vi "Custom Device CORE.vi"(8 "error in (no error)":errorcluster, 11 "CDW_MetaDataObj":refnum<class "NIVS_Consolidated_CDW_MetaDataObj.lvclass">) -> (0 "error out":errorcluster)   [LabVIEW 2015, in "NIVS_Consolidated_CDW_MetaDataObj.lvclass"]
doc: "This VI is the Core VI for the Custom Device Wizard.\n\nWritten by:\nStephan Daunke\n\nDate:\n2014/01/27\n\nCompany:\nNational Instruments Germany GmbH"
uses:
  NIVS_Consolidated_CDW_MetaDataObj.lvclass
  Action.ctl
  Internal data.ctl
  <resource>/dialog/NewProjectWizard/MetaDataObj/MetaDataObj.lvclass/MetaDataObj.ctl
  NIVS_Consolidated_CDW_MetaDataObj.lvclass/NIVS_Consolidated_CDW_MetaDataObj.ctl
  Template Classes/NIVS_CD Template/NIVS_CD Template.lvclass/NIVS_CD Template.ctl
  Utility folder.ctl
  CD Shared lvlib.ctl
  Common.ctl
  Add Item - Type.ctl
  CD System Explorer lvlib.ctl
  <vilib>/Utility/traverseref.llb/TRef TravTarget.ctl
  CD Engine lvlib.ctl
  Build Spec System Explorer.ctl
  Build Spec Engine.ctl
  <resource>/dialog/NewProjectWizard/MetaDataObj/Accessors/Read Project Root.vi
  Read CD Template.vi
  Template Classes/NIVS_CD Template/Read Extra Page Names.vi
  <resource>/dialog/NewProjectWizard/MetaDataObj/Accessors/Read Project Name.vi
  Utility folder.vi
  CD Shared lvlib.vi
  Common.vi
  CD System Explorer lvlib.vi
  CD Engine lvlib.vi
  <vilib>/Utility/config.llb/Write Key (String).vi
  <vilib>/Utility/config.llb/Write Key (Path).vi
  Build Spec System Explorer.vi
  Build Spec Engine.vi
  Template Classes/NIVS_CD Template/NIVS_CD Template.lvclass
  <vilib>/Utility/config.llb/NI_LVConfig.lvlib
  <vilib>/Utility/Data Type/NI_Data Type.lvlib
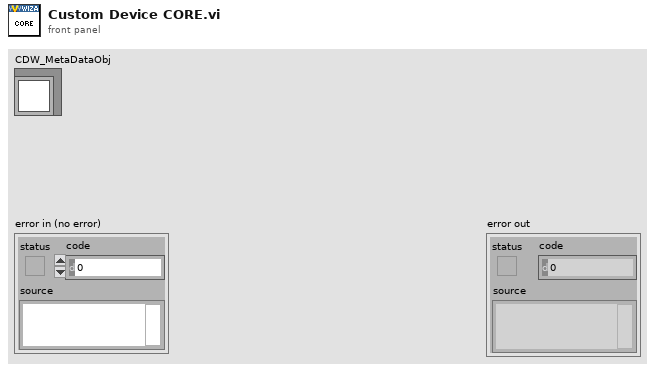
[diagram p1: front panel]
types:
  T1 = typedef "NIVS_Consolidated_CDW_MetaDataObj.lvclass/Internal data.ctl" = cluster{"CD GUID":string, "Extra Page GUIDs":string[], "System Explorer Library":refnum<vi>, "Shared Library":refnum<vi>, "Engine Library":refnum<vi>}
  T2 = typedef "NIVS_Consolidated_CDW_MetaDataObj.lvclass/Action.ctl" = enum16{"Project - Create Custom Device folder", "PC - Create GUID for each extra page", "PC-Utility - Create folder and copy -Copy .LLB to NI VeriStand dir-", "PC-Utility - Change -Copy .LLB to NI VeriStand dir-", "PC-Shared - Create folder and copy Constants.vi", "PC-Shared - Change Constants.vi content", "PC-Shared - Create library", "PC-Shared - Add folders and VIs to library", "PC-System Explorer - Create folder and copy templates", "PC-System Explorer - Create extra pages", "PC-System Explorer - Create library", "PC-System Explorer - Add folders and VIs to library", "PC-Engine - Create folder and copy the RT Template", "PC-Engine - Create library", "PC-Engine - Add virtual folders and VIs to library", "PC-XML - Create and change file", "PC-Help - Copy HTML Files", "Project - Read project file content", "Project - Edit Utility section", "Project - Edit XML section", "Project - Edit Engine Library section", "Project - Edit Shared Library section", "Project - Edit System Explorer Library section", "Project - Edit Custom Device Name", "Project - Edit System Explorer LLB Name", "Project - Edit Engine LLB OS dependent file name", "Project - Write new project file"}
  T3 = typedef "NIVS_Consolidated_CDW_MetaDataObj.lvclass/Utility folder.ctl" = enum16{"Utility.FolderName", "Utility.Copy .llb to NI VeriStand dir.FileName", "Utility.Copy .llb to NI VeriStand dir.FilePathAndName", "Utility.LLB Pre Build.FilePathAndName"}
  T4 = typedef "NIVS_Consolidated_CDW_MetaDataObj.lvclass/CD Shared lvlib.ctl" = enum16{"LibraryFileName", "LibraryFolderName", "ConstantsVI.VIPathAndName", "Shared.FolderName", "Shared.Types.FolderName", "Shared.Constants.VIName", "Shared.Constants.VITemplateName", "Shared.Constants.VITemplatePathAndName", "Shared.CompiledSettings.RelativePath", "Shared.Constants.RelativePath", "Shared.CompiledSettings.Name", "Shared.CompiledSettings.Name.NoExtension", "Shared.CompiledSettings.ClusterName"}
  T5 = typedef "NIVS_Consolidated_CDW_MetaDataObj.lvclass/Common.ctl" = enum16{"ProjectName", "TemplatesFolderName", "ProjectTemplatePathAndName", "TimingAndSyncFolderName", "CustomDeviceFolderName", "PathToTemplates"}
  T6 = typedef "NIVS_Consolidated_CDW_MetaDataObj.lvclass/Add Item - Type.ctl" = string
  T7 = typedef "NIVS_Consolidated_CDW_MetaDataObj.lvclass/CD System Explorer lvlib.ctl" = enum16{"LibraryFileName", "LibraryFolderName", "System Explorer.FolderName", "System Explorer.Dynamically Called.FolderName", "System Explorer.Dynamically Called.Extra Pages.FolderName", "System Explorer.Dynamically Called.Extra Pages.TemplatePathAndName", "System Explorer.Dynamically Called.Main Page.VIName", "System Explorer.Dynamically Called.Main Page.TemplatePathAndName", "System Explorer.Dynamically Called.Initialization VI.VIName", "System Explorer.Dynamically Called.Initialization VI.TemplatePathAndName", "System Explorer.SubVI.FolderName", "System Explorer.Types.FolderName", "System Explorer.ActionVIOnCompile.VIName", "System Explorer.ExportConfigRTM.VIName", "System Explorer.LoadHelpFile.VIName"}
  T8 = typedef "TRef TravTarget.ctl" = enum16{"FP", "BD", "Other"}
  T9 = typedef "NIVS_Consolidated_CDW_MetaDataObj.lvclass/CD Engine lvlib.ctl" = enum16{"LibraryFileName", "LibraryFolderName", "Engine.FolderName", "Engine.Init.FolderName", "Engine.Run.FolderName", "Engine.Shutdown.FolderName", "Types.FolderName", "Engine.RT Driver VI.TemplatePath", "Engine.RT Driver VI.FileName", "Engine.RTStateVariables.Name", "Engine.RTStateVariables.Name.NoExtension", "Engine.Async.NameExtension", "Engine.Async.TemplateName"}
  T10 = typedef "NIVS_Consolidated_CDW_MetaDataObj.lvclass/Build Spec System Explorer.ctl" = enum16{"Destinations.LLBFileName"}
  T11 = typedef "NIVS_Consolidated_CDW_MetaDataObj.lvclass/Build Spec Engine.ctl" = enum16{"Destinations.LLBWindowsFileName", "Destinations.LLBVxWorksFileName", "Destinations.LLBPharlapFileName", "Destinations.LLBLinuxARMFileName", "Destinations.LLBLinux64FileName"}
  T12 = enum16{"open", "replace", "create", "open or create", "replace or create", "replace or create with confirmation"}
  T13 = typedef "NI_LVConfig.lvlib/Config Data RefNum.ctl" = refnum<k1>
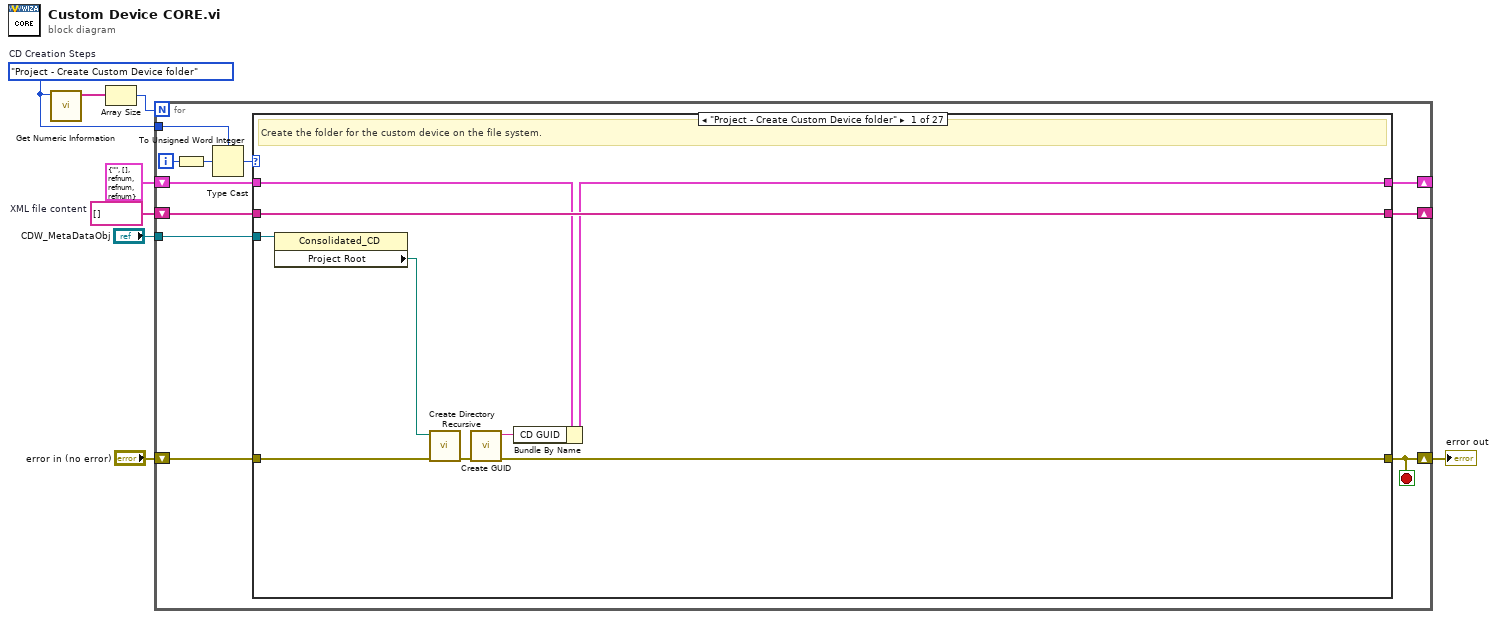
[diagram p0: block diagram]
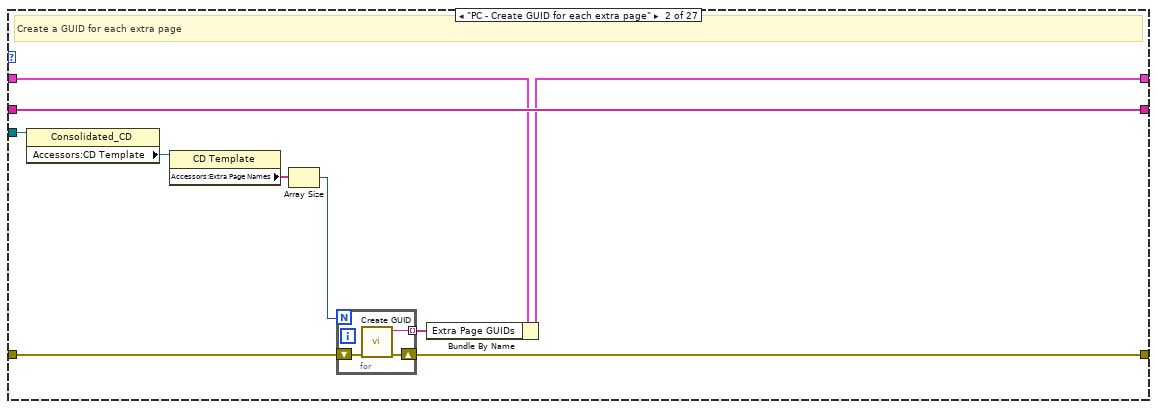
[diagram p2: hidden frame]
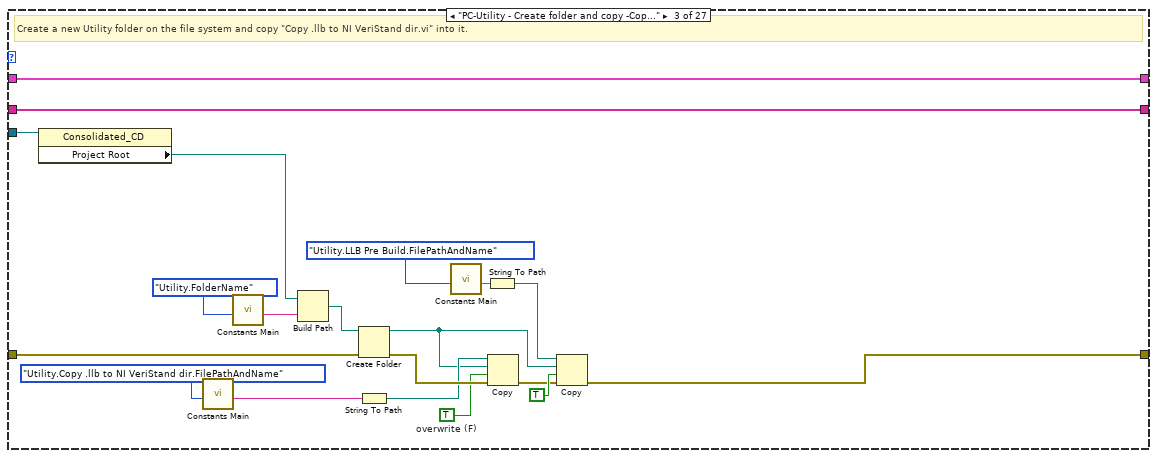
[diagram p3: hidden frame]
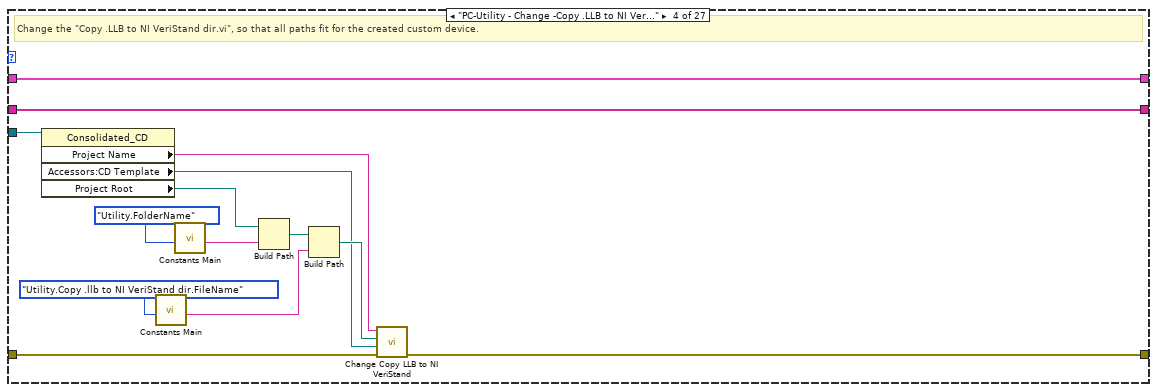
[diagram p4: hidden frame]
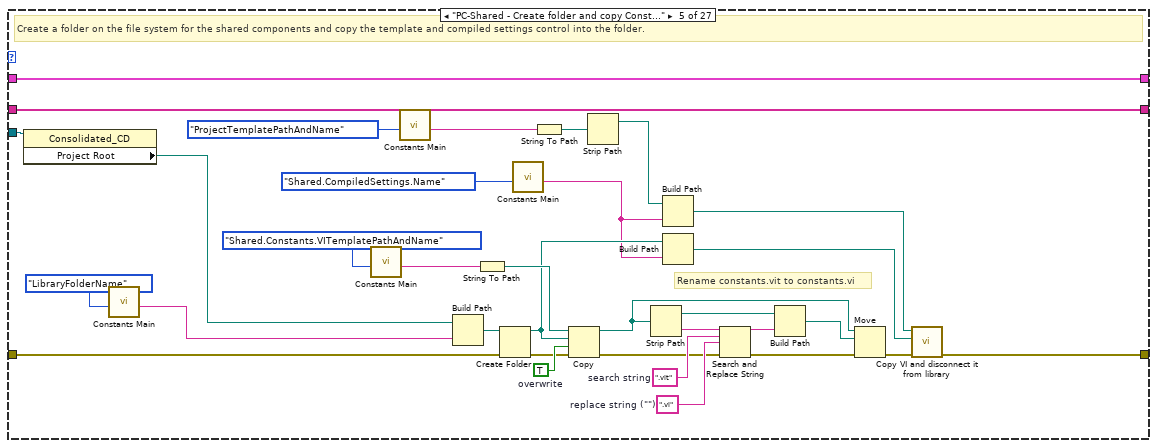
[diagram p5: hidden frame]
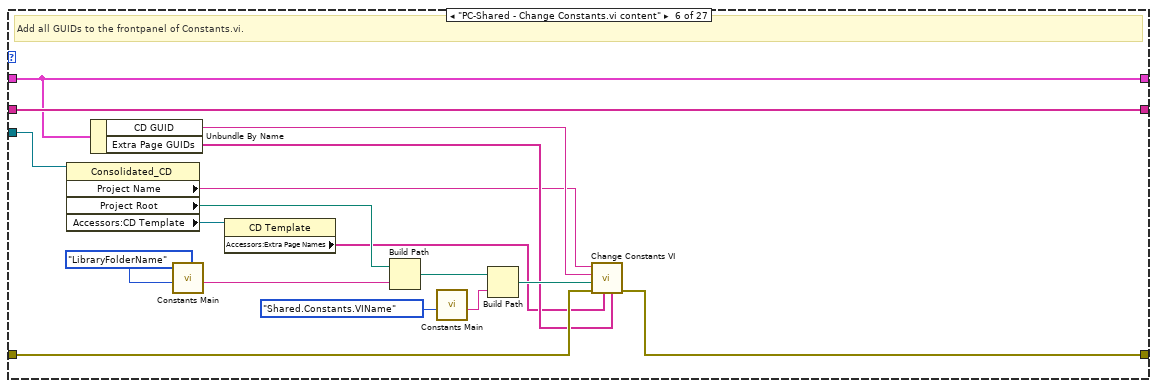
[diagram p6: hidden frame]
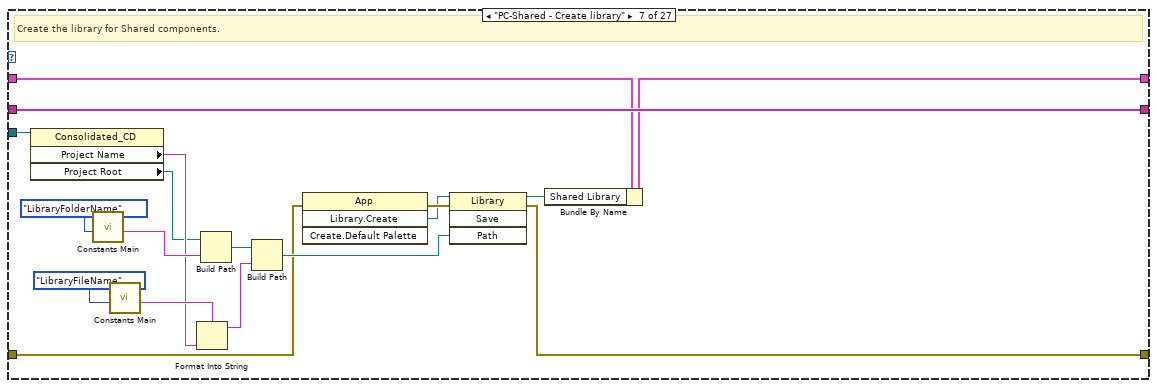
[diagram p7: hidden frame]
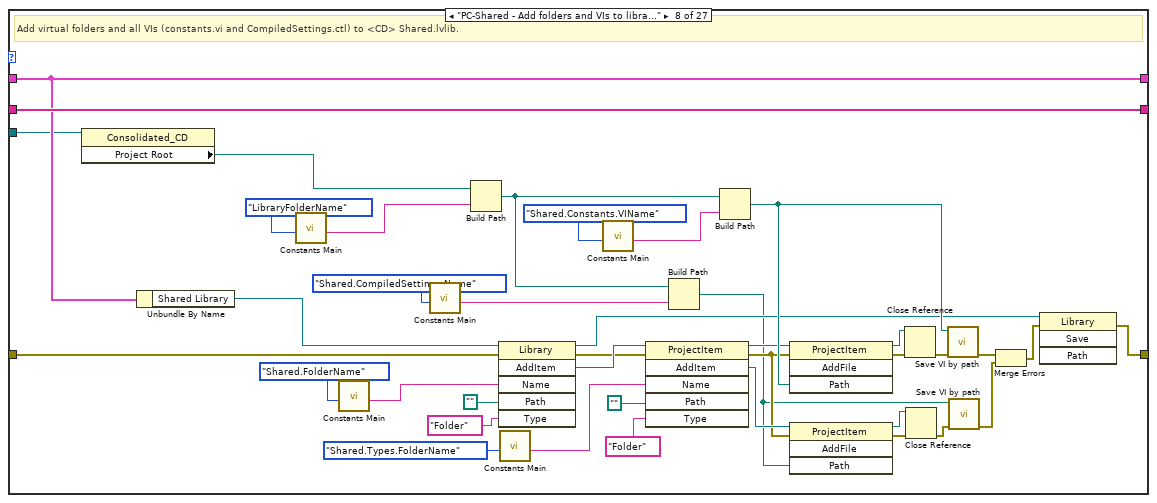
[diagram p8: hidden frame]
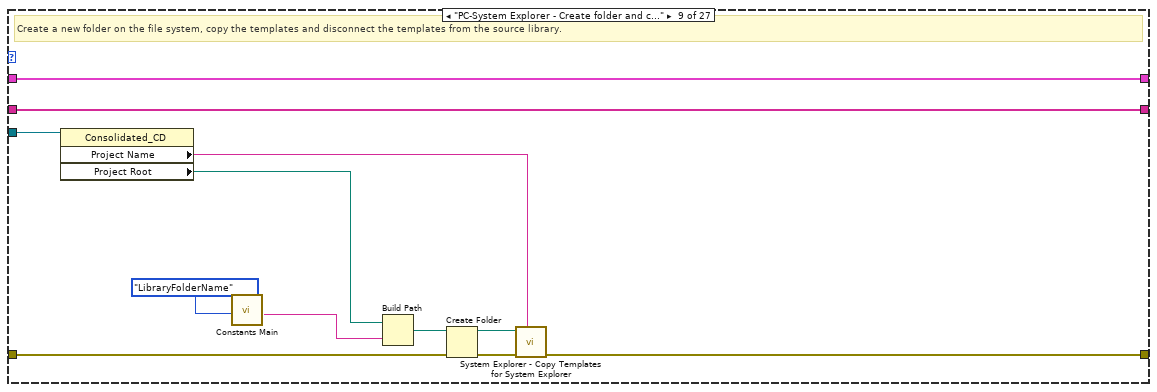
[diagram p9: hidden frame]
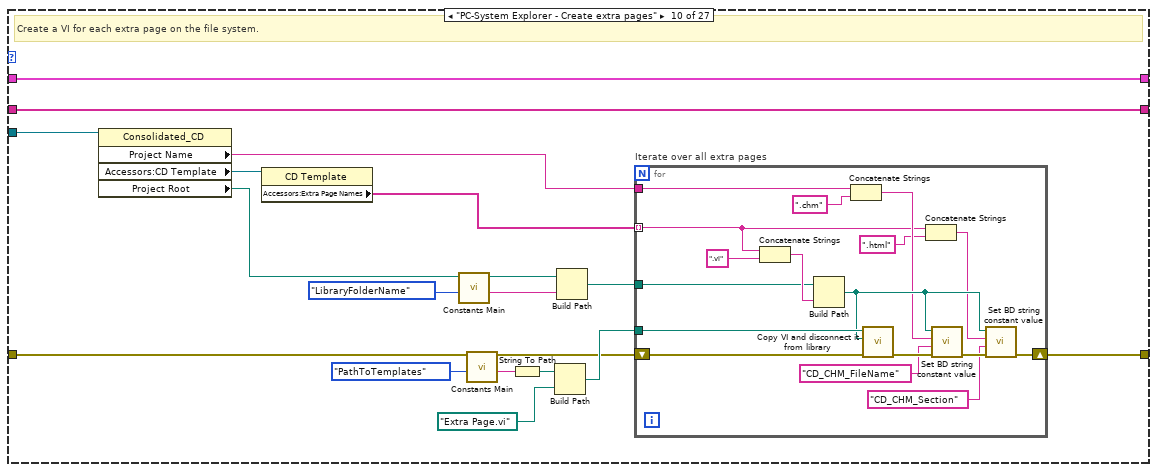
[diagram p10: hidden frame]
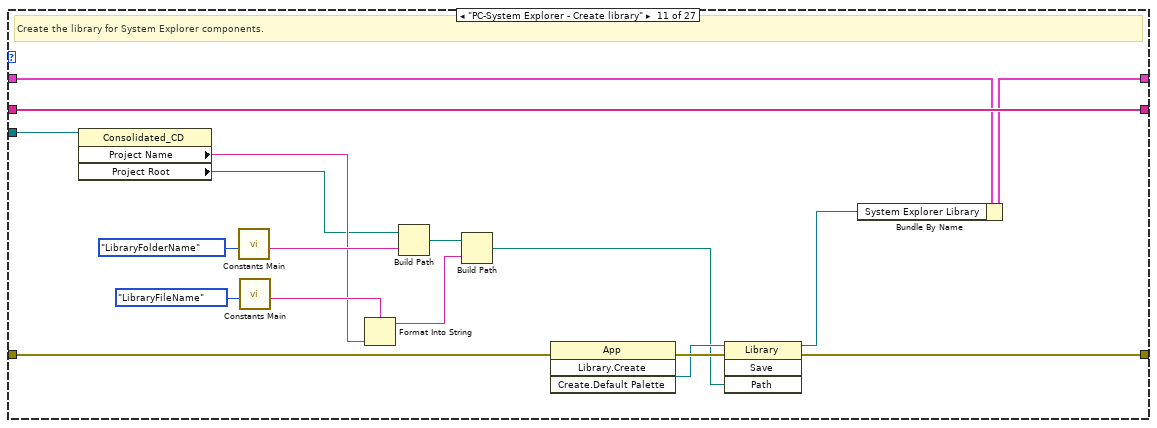
[diagram p11: hidden frame]
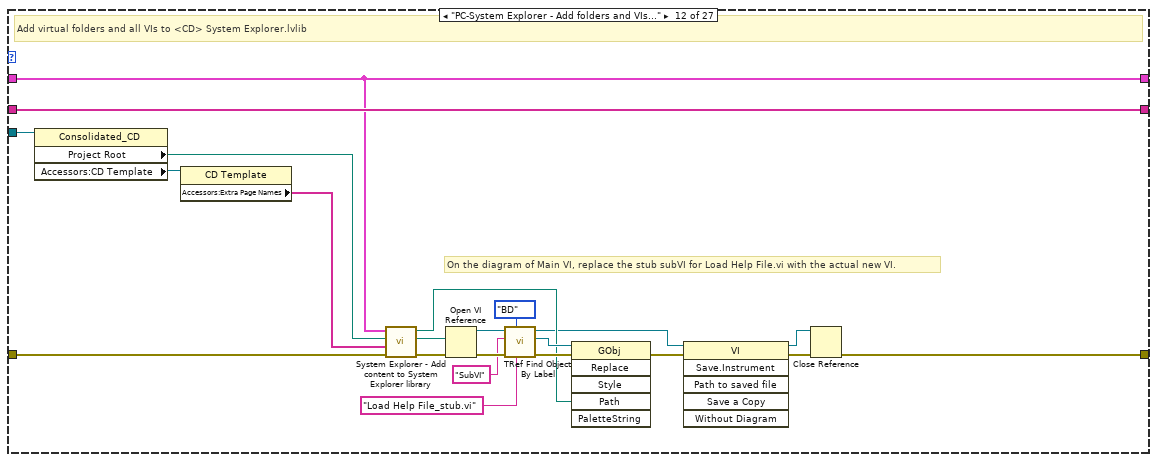
[diagram p12: hidden frame]
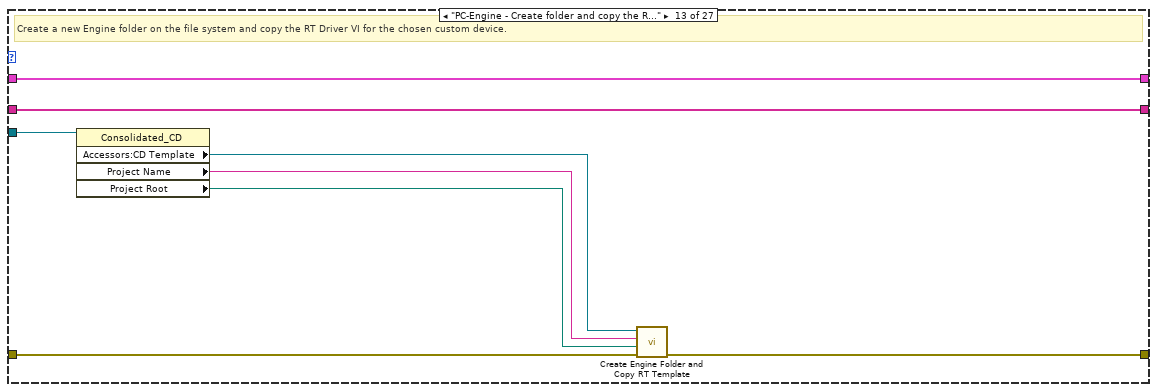
[diagram p13: hidden frame]
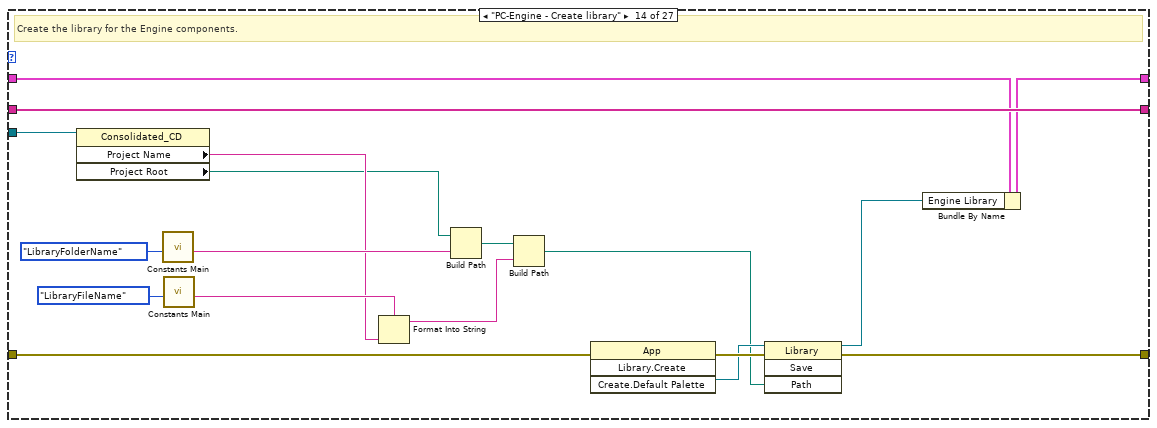
[diagram p14: hidden frame]
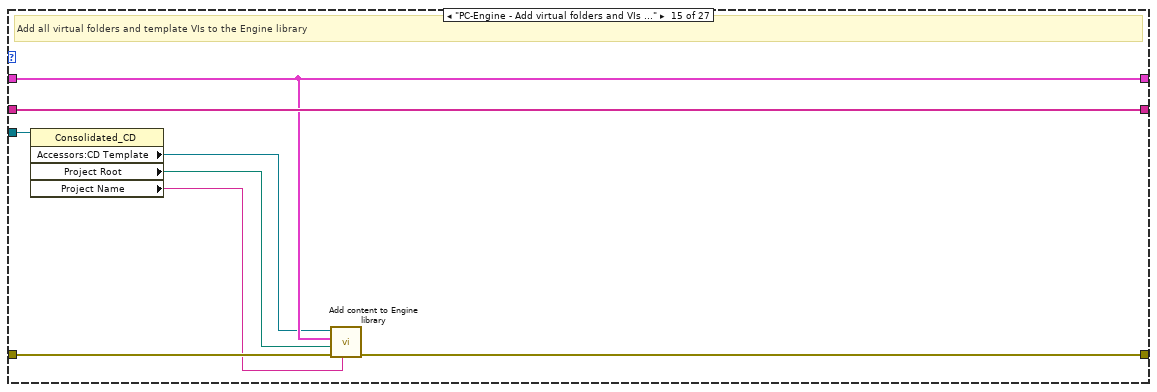
[diagram p15: hidden frame]
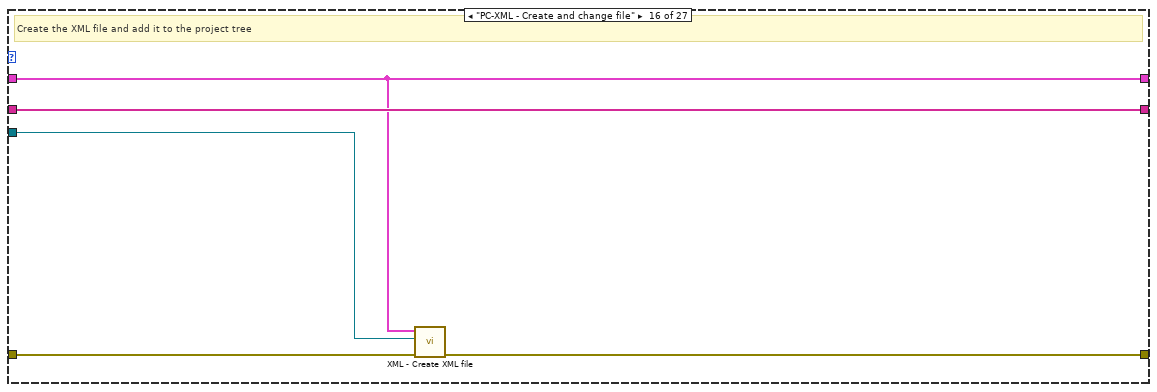
[diagram p16: hidden frame]
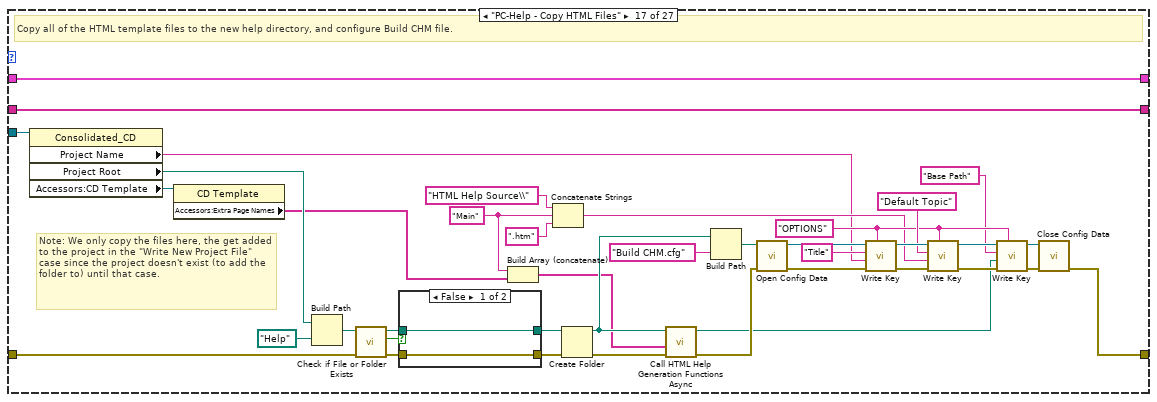
[diagram p17: hidden frame]
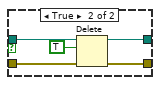
[diagram p18: hidden frame]
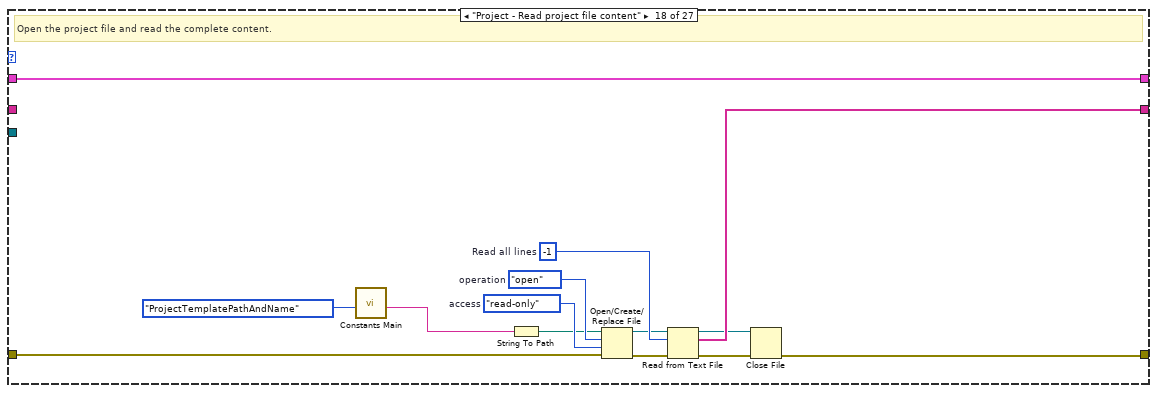
[diagram p19: hidden frame]
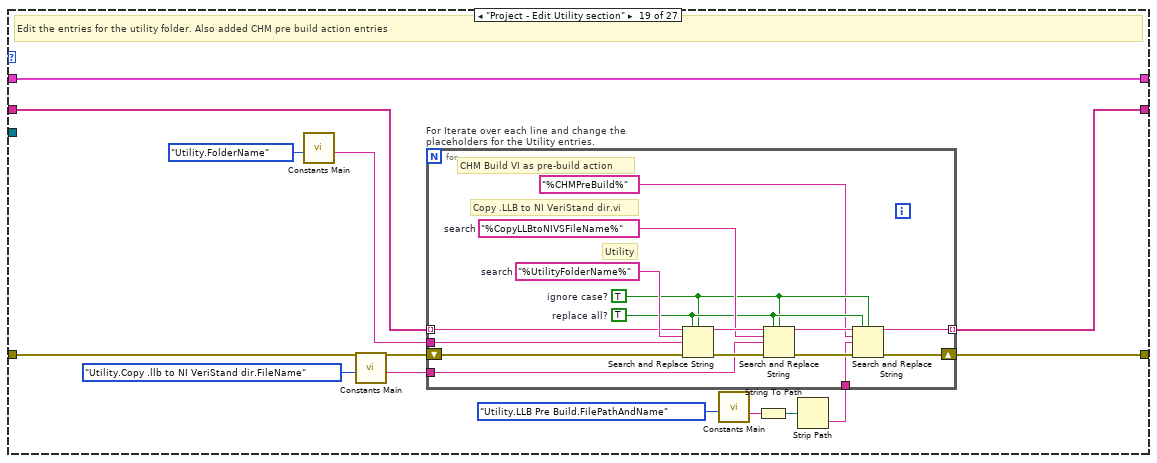
[diagram p20: hidden frame]
diagram:
  w4 = Action."Project - Create Custom Device folder"  # CD Creation Steps
  w5 = string[] []  # XML file content
  n1 = call <vilib>:"Get Numeric Information.vi"("Variant"=w4) -> ("Enum Names"=w3:string[])  [unwired: 7 in, 3 out]
  n2 = Array Size(array=w3) -> (size(s)=w2:i32)
  n3 = for {
    N: w2 -> [_]
    shift-right: [w16] -> _
    shift-left: T1 {"CD GUID"="", "Extra Page GUIDs"=[], "System Explorer Library"=refnum, "Shared Library"=refnum, "Engine Library"=refnum} ("CD Wizard - Internal Data") -> [w18]
    shift-right: [w15] -> _
    shift-left: w5 -> [w17]
    shift-right: [w14] -> w6
    shift-left: "error in (no error)" -> [w19]
    tunnel: w4 -> [w12]
    tunnel: "CDW_MetaDataObj" -> [w11]
    i -> [w13]
    stop <- w14 stop-if-true
    n4 = To Unsigned Word Integer(number=w13) -> (unsigned 16bit integer=w9:u16)
    n5 = Type Cast(type=w12, x=w9) -> (*(type *) &x=w10:T2)
    n6 = case shown="\"Project - Create Custom Device folder\"" w10 {
      tunnel: w19 -> [w24 w37 w43 w63 w78 w118 w129 w145 w183 w200 w232 w267 w275 w280 w301 w306 w324 w354 w367 w399 w418 w422 w452 w486 w497 w515 w553]
      tunnel: [w25 w36 w47 w69 w80 w124 w130 w163 w188 w210 w233 w252 w274 w283 w300 w305 w323 w360 w376 w404 w417 w432 w456 w485 w504 w527 w560] -> w14
      tunnel: w18 -> [w22 w34 w46 w67 w79 w115 w133 w164 w187 w209 w238 w265 w273 w287 w298 w304 w319 w366 w379 w401 w416 w423 w453 w482 w501 w533 w585]
      tunnel: w17 -> [w28 w38 w61 w75 w108 w125 w143 w182 w194 w211 w246 w268 w276 w294 w302 w307 w346 _ w378 w403 w415 w427 w454 w483 w499 w528 w579]
      tunnel: [w27 w33 w46 w67 w79 w115 w132 w164 w187 w209 w239 w265 w273 w286 w298 w304 w319 w366 w379 w401 w416 w423 w453 w482 w501 w533 w585] -> w16
      tunnel: [w28 w38 w61 w75 w108 w125 w143 w182 w194 w211 w246 w268 w276 w294 w302 w307 w346 w359 w377 w402 w419 w433 w455 w484 w498 w516 w579] -> w15
      tunnel: w11 -> [w21 w32 w45 w66 w77 w117 w128 w147 w186 w199 w231 w250 w272 w279 w299 w303 w312 _ _ w398 w414 w421 w451 w481 w496 w514 w552]
      frame "Project - Create Custom Device folder" {
        # "Create the folder for the custom device on the file system."
        n7 = property class="Consolidated_CD"(reference=w21) -> ("Project Root"=w20:path)  [unwired: 1 in, 2 out]
        n8 = call <vilib>:"Create Directory Recursive.vi"("error in (no error)"=w24, "directory"=w20) -> ("error out"=w23:errorcluster)  [unwired: 3 in, 2 out]
        n9 = call "Create GUID.vi"("error in (no error)"=w23) -> ("error out"=w25:errorcluster, "Generated GUID"=w26:string)  [unwired: 9 in]
        n10 = Bundle By Name(cluster=w22, "CD GUID"=w26) -> (w27:T1)
      }
      frame "PC - Create GUID for each extra page" {
        # "Create a GUID for each extra page"
        n11 = property class="Consolidated_CD"(reference=w32) -> ("Accessors:CD Template"=w31:refnum<class "NIVS_CD Template.lvclass">)  [unwired: 1 in, 2 out]
        n12 = property class="CD Template"(reference=w31) -> ("Accessors:Extra Page Names"=w30:string[])  [unwired: 1 in, 2 out]
        n13 = Array Size(array=w30) -> (size(s)=w29:i32)
        n14 = for {
          N: w29 -> [_]
          shift-right: [w40] -> w36
          shift-left: w37 -> [w41]
          tunnel: [w39] -> w35 mode=indexing
          n15 = call "Create GUID.vi"("error in (no error)"=w41) -> ("error out"=w40:errorcluster, "Generated GUID"=w39:string)  [unwired: 9 in]
        }
        n16 = Bundle By Name(cluster=w34, "Extra Page GUIDs"=w35) -> (w33:T1)
      }
      frame "PC-Utility - Create folder and copy -Copy .LLB to NI VeriStand dir-" {
        w58 = TRUE  # overwrite (F)
        # "Create a new Utility folder on the file system and copy \"Copy .llb to NI VeriStand dir.vi\" into it."
        n17 = property class="Consolidated_CD"(reference=w45) -> ("Project Root"=w44:path)  [unwired: 1 in, 2 out]
        n18 = call-poly "Constants Main.vi"("Action"=Utility_folder."Utility.Copy .llb to NI VeriStand dir.FilePathAndName") -> ("Output"=w56:string)  [unwired: 10 in]
        n19 = call-poly "Constants Main.vi"("Action"=Utility_folder."Utility.FolderName") -> ("Output"=w53:string)  [unwired: 10 in]
        n20 = Build Path(base path=w44, name or relative path=w53) -> (appended path=w60:path)
        n21 = Create Folder(path (use dialog)=w60, error in=w43) -> (created path=w52:path, error out=w59:errorcluster)  [unwired: 1 in, 1 out]
        n22 = String To Path(string=w56) -> (path=w55:path)
        n23 = call-poly "Constants Main.vi"("Action"=Utility_folder."Utility.LLB Pre Build.FilePathAndName") -> ("Output"=w50:string)  [unwired: 10 in]
        n24 = String To Path(string=w50) -> (path=w49:path)
        n25 = Copy(8:w59, 9:w58, 10:w52, 11:w55) -> (0:w42:errorcluster)  [unwired: 3 out]
        n26 = Copy(8:w42, 9:TRUE ("overwrite (F)"), 10:w52, 11:w49) -> (0:w47:errorcluster)  [unwired: 3 out]
      }
      frame "PC-Utility - Change -Copy .LLB to NI VeriStand dir-" {
        # "Change the \"Copy .LLB to NI VeriStand dir.vi\", so that all paths fit for the created custom device."
        n27 = property class="Consolidated_CD"(reference=w66) -> ("Project Name"=w65:string, "Accessors:CD Template"=w64:refnum<class "NIVS_CD Template.lvclass">, "Project Root"=w62:path)  [unwired: 1 in, 2 out]
        n28 = call-poly "Constants Main.vi"("Action"=Utility_folder."Utility.Copy .llb to NI VeriStand dir.FileName") -> ("Output"=w70:string)  [unwired: 10 in]
        n29 = call-poly "Constants Main.vi"("Action"=Utility_folder."Utility.FolderName") -> ("Output"=w72:string)  [unwired: 10 in]
        n30 = Build Path(base path=w62, name or relative path=w72) -> (appended path=w71:path)
        n31 = Build Path(base path=w71, name or relative path=w70) -> (appended path=w68:path)
        n32 = call "Change Copy LLB to NI VeriStand.vi"("error in (no error)"=w63, "CD Template"=w64, "Copy .LLB to ... path"=w68, "CD Name"=w65) -> ("error out"=w69:errorcluster)  [unwired: 7 in]
      }
      frame "PC-Shared - Create folder and copy Constants.vi" {
        w97 = ".vi"  # replace string ("")
        w98 = ".vit"  # search string
        w102 = TRUE  # overwrite
        # "Rename constants.vit to constants.vi"
        # "Create a folder on the file system for the shared components and copy the template and compiled settings control into the folder."
        n33 = property class="Consolidated_CD"(reference=w77) -> ("Project Root"=w76:path)  [unwired: 1 in, 2 out]
        n34 = call-poly "Constants Main.vi"("Action"=CD_Shared_lvlib."LibraryFolderName") -> ("Output"=w105:string)  [unwired: 10 in]
        n35 = call-poly "Constants Main.vi"("Action"=CD_Shared_lvlib."Shared.Constants.VITemplatePathAndName") -> ("Output"=w103:string)  [unwired: 10 in]
        n36 = call-poly "Constants Main.vi"("Action"=Common."ProjectTemplatePathAndName") -> ("Output"=w89:string)  [unwired: 10 in]
        n37 = Build Path(base path=w76, name or relative path=w105) -> (appended path=w107:path)
        n38 = String To Path(string=w103) -> (path=w95:path)
        n39 = Create Folder(path (use dialog)=w107, error in=w78) -> (created path=w86:path, error out=w96:errorcluster)  [unwired: 1 in, 1 out]
        n40 = call-poly "Constants Main.vi"("Action"=CD_Shared_lvlib."Shared.CompiledSettings.Name") -> ("Output"=w81:string)  [unwired: 10 in]
        n41 = String To Path(string=w89) -> (path=w88:path)
        n42 = Copy(8:w96, 9:w102, 10:w86, 11:w95) -> (0:w94:errorcluster, 3:w91:path)  [unwired: 2 out]
        n43 = Strip Path(path=w88) -> (stripped path=w87:path)  [unwired: 1 out]
        n44 = Strip Path(path=w91) -> (stripped path=w101:path, name=w100:string)
        n45 = Build Path(base path=w87, name or relative path=w81) -> (appended path=w85:path)
        n46 = Build Path(base path=w86, name or relative path=w81) -> (appended path=w84:path)
        n47 = Search and Replace String(input string=w100, search string=w98, replace string=w97, error in=w94) -> (result string=w99:string, error out=w93:errorcluster)  [unwired: 4 in, 2 out]
        n48 = Build Path(base path=w101, name or relative path=w99) -> (appended path=w92:path)
        n49 = Move(source path=w91, error in=w93, 10:w92) -> (error out=w83:errorcluster)  [unwired: 2 in, 2 out]
        n50 = call "Copy VI and disconnect it from library.vi"("error in (no error)"=w83, "VI Target Path"=w84, "VI Source Path"=w85) -> ("error out"=w80:errorcluster)  [unwired: 8 in]
      }
      frame "PC-Shared - Change Constants.vi content" {
        # "Add all GUIDs to the frontpanel of Constants.vi."
        n51 = property class="Consolidated_CD"(reference=w117) -> ("Project Name"=w111:string, "Project Root"=w116:path, "Accessors:CD Template"=w110:refnum<class "NIVS_CD Template.lvclass">)  [unwired: 1 in, 2 out]
        n52 = Unbundle By Name(w115) -> ("CD GUID"=w113:string, "Extra Page GUIDs"=w112:string[])
        n53 = call-poly "Constants Main.vi"("Action"=CD_Shared_lvlib."LibraryFolderName") -> ("Output"=w119:string)  [unwired: 10 in]
        n54 = property class="CD Template"(reference=w110) -> ("Accessors:Extra Page Names"=w109:string[])  [unwired: 1 in, 2 out]
        n55 = Build Path(base path=w116, name or relative path=w119) -> (appended path=w123:path)
        n56 = call-poly "Constants Main.vi"("Action"=CD_Shared_lvlib."Shared.Constants.VIName") -> ("Output"=w121:string)  [unwired: 10 in]
        n57 = Build Path(base path=w123, name or relative path=w121) -> (appended path=w114:path)
        n58 = call "Change Constants VI.vi"("Extra Page GUIDs"=w112, "Extra Page Names"=w109, "error in (no error)"=w118, "Constants.vi path"=w114, "CD GUID"=w113, "CD Name"=w111) -> ("error out"=w124:errorcluster)  [unwired: 5 in]
      }
      frame "PC-Shared - Create library" {
        # "Create the library for Shared components."
        n59 = property class="Consolidated_CD"(reference=w128) -> ("Project Name"=w127:string, "Project Root"=w126:path)  [unwired: 1 in, 2 out]
        n60 = call-poly "Constants Main.vi"("Action"=CD_Shared_lvlib."LibraryFolderName") -> ("Output"=w137:string)  [unwired: 10 in]
        n61 = call-poly "Constants Main.vi"("Action"=CD_Shared_lvlib."LibraryFileName") -> ("Output"=w138:string)  [unwired: 10 in]
        n62 = Format Into String(format string=w138, w127) -> (resulting string=w141:string)  [unwired: 2 in, 1 out]
        n63 = Build Path(base path=w126, name or relative path=w137) -> (appended path=w142:path)
        n64 = Build Path(base path=w142, name or relative path=w141) -> (appended path=w134:path)
        n65 = invoke class="App" method="Library.Create"(error in=w129) -> (error out=w136:errorcluster, "Create Library"=w135:refnum<vi>)  [unwired: 3 in, 2 out]
        n66 = invoke class="Library" method="Save"(reference=w135, error in=w136, "Path"=w134) -> (reference out=w131:refnum<vi>, error out=w130:errorcluster)  [unwired: 1 in, 2 out]
        n67 = Bundle By Name(cluster=w133, "Shared Library"=w131) -> (w132:T1)
      }
      frame "PC-Shared - Add folders and VIs to library" {
        # "Add virtual folders and all VIs (constants.vi and CompiledSettings.ctl) to <CD> Shared.lvlib."
        n68 = property class="Consolidated_CD"(reference=w147) -> ("Project Root"=w146:path)  [unwired: 1 in, 2 out]
        n69 = Unbundle By Name(w164) -> ("Shared Library"=w166:refnum<vi>)
        n70 = call-poly "Constants Main.vi"("Action"=CD_Shared_lvlib."LibraryFolderName") -> ("Output"=w160:string)  [unwired: 10 in]
        n71 = call-poly "Constants Main.vi"("Action"=CD_Shared_lvlib."Shared.FolderName") -> ("Output"=w161:string)  [unwired: 10 in]
        n72 = call-poly "Constants Main.vi"("Action"=CD_Shared_lvlib."Shared.CompiledSettings.Name") -> ("Output"=w152:string)  [unwired: 10 in]
        n73 = Build Path(base path=w146, name or relative path=w160) -> (appended path=w157:path)
        n74 = invoke class="Library" method="AddItem"(reference=w166, error in=w145, "Name"=w161, "Path"=path "", "Type"=T6 "Folder" ("Add Item - Type")) -> (reference out=w172:refnum<vi>, error out=w167:errorcluster, "AddItem"=w169:refnum<vi>)  [unwired: 1 in, 3 out]
        n75 = call-poly "Constants Main.vi"("Action"=CD_Shared_lvlib."Shared.Types.FolderName") -> ("Output"=w180:string)  [unwired: 10 in]
        n76 = call-poly "Constants Main.vi"("Action"=CD_Shared_lvlib."Shared.Constants.VIName") -> ("Output"=w148:string)  [unwired: 10 in]
        n77 = invoke class="ProjectItem" method="AddItem"(reference=w169, error in=w167, "Name"=w180, "Path"=path "", "Type"=T6 "Folder" ("Add Item - Type")) -> (reference out=w171:refnum<vi>, error out=w158:errorcluster, "AddItem"=w159:refnum<vi>)  [unwired: 1 in, 3 out]
        n78 = Build Path(base path=w157, name or relative path=w152) -> (appended path=w156:path)
        n79 = Build Path(base path=w157, name or relative path=w148) -> (appended path=w173:path)
        n80 = invoke class="ProjectItem" method="AddFile"(reference=w171, error in=w158, "Path"=w173) -> (reference out=w176:refnum<vi>, error out=w175:errorcluster)  [unwired: 1 in, 2 out]
        n81 = invoke class="ProjectItem" method="AddFile"(reference=w159, error in=w158, "Path"=w156) -> (reference out=w150:refnum<vi>, error out=w149:errorcluster)  [unwired: 1 in, 2 out]
        n82 = Close Reference(reference=w176, error in (no error)=w175) -> (error out=w177:errorcluster)
        n83 = Close Reference(reference=w150, error in (no error)=w149) -> (error out=w151:errorcluster)
        n84 = call "Save VI by path.vi"("error in (no error)"=w177, "VI path"=w173) -> ("error out"=w174:errorcluster)  [unwired: 9 in]
        n85 = call "Save VI by path.vi"("error in (no error)"=w151, "VI path"=w156) -> ("error out"=w154:errorcluster)  [unwired: 9 in]
        n86 = Merge Errors(w174, w154) -> (w155:errorcluster)
        n87 = invoke class="Library" method="Save"(reference=w172, error in=w155) -> (error out=w163:errorcluster)  [unwired: 2 in, 3 out]
      }
      frame "PC-System Explorer - Create folder and copy templates" {
        # "Create a new folder on the file system, copy the templates and disconnect the templates from the source library."
        n88 = property class="Consolidated_CD"(reference=w186) -> ("Project Name"=w185:string, "Project Root"=w184:path)  [unwired: 1 in, 2 out]
        n89 = call-poly "Constants Main.vi"("Action"=CD_System_Explorer_lvlib."LibraryFolderName") -> ("Output"=w191:string)  [unwired: 10 in]
        n90 = Build Path(base path=w184, name or relative path=w191) -> (appended path=w193:path)
        n91 = Create Folder(path (use dialog)=w193, error in=w183) -> (created path=w189:path, error out=w190:errorcluster)  [unwired: 1 in, 1 out]
        n92 = call "System Explorer - Copy Templates for System Explorer.vi"("CD Name"=w185, "error in (no error)"=w190, "System Explorer folder"=w189) -> ("error out"=w188:errorcluster)  [unwired: 8 in]
      }
      frame "PC-System Explorer - Create extra pages" {
        # "Create a VI for each extra page on the file system."
        n93 = property class="Consolidated_CD"(reference=w199) -> ("Project Name"=w198:string, "Accessors:CD Template"=w197:refnum<class "NIVS_CD Template.lvclass">, "Project Root"=w195:path)  [unwired: 1 in, 2 out]
        n94 = property class="CD Template"(reference=w197) -> ("Accessors:Extra Page Names"=w196:string[])  [unwired: 1 in, 2 out]
        n95 = call-poly "Constants Main.vi"("Action"=CD_System_Explorer_lvlib."LibraryFolderName") -> ("Output"=w207:string)  [unwired: 10 in]
        n96 = call-poly "Constants Main.vi"("Action"=Common."PathToTemplates") -> ("Output"=w203:string)  [unwired: 10 in]
        n97 = String To Path(string=w203) -> (path=w202:path)
        n98 = Build Path(base path=w202, name or relative path=path "Extra Page.vi") -> (appended path=w208:path)
        n99 = Build Path(base path=w195, name or relative path=w207) -> (appended path=w205:path)
        n100 = for "Iterate over all extra pages" {
          tunnel: w196 -> [w212] mode=indexing
          shift-right: [w217] -> w210
          shift-left: w200 -> [w226]
          tunnel: w205 -> [w224]
          tunnel: w208 -> [w225]
          tunnel: w198 -> [w221]
          n101 = Concatenate Strings(w212, ".vi") -> (w227:string)
          n102 = Build Path(base path=w224, name or relative path=w227) -> (appended path=w219:path)
          n103 = Concatenate Strings(w221, ".chm" ("string")) -> (w216:string)
          n104 = call "Copy VI and disconnect it from library.vi"("error in (no error)"=w226, "VI Target Path"=w219, "VI Source Path"=w225) -> ("error out"=w223:errorcluster)  [unwired: 8 in]
          n105 = Concatenate Strings(w212, ".html" ("string")) -> (w214:string)
          n106 = call "Set BD string constant value.vi"("error in (no error)"=w223, "Name of string constant"="CD_CHM_FileName", "New String Value"=w216, "Path to VI"=w219) -> ("error out"=w220:errorcluster)  [unwired: 7 in]
          n107 = call "Set BD string constant value.vi"("error in (no error)"=w220, "Name of string constant"="CD_CHM_Section", "New String Value"=w214, "Path to VI"=w219) -> ("error out"=w217:errorcluster)  [unwired: 7 in]
        }
      }
      frame "PC-System Explorer - Create library" {
        # "Create the library for System Explorer components."
        n108 = property class="Consolidated_CD"(reference=w231) -> ("Project Name"=w230:string, "Project Root"=w229:path)  [unwired: 1 in, 2 out]
        n109 = call-poly "Constants Main.vi"("Action"=CD_System_Explorer_lvlib."LibraryFolderName") -> ("Output"=w242:string)  [unwired: 10 in]
        n110 = call-poly "Constants Main.vi"("Action"=CD_System_Explorer_lvlib."LibraryFileName") -> ("Output"=w243:string)  [unwired: 10 in]
        n111 = Format Into String(format string=w243, w230) -> (resulting string=w244:string)  [unwired: 2 in, 1 out]
        n112 = Build Path(base path=w229, name or relative path=w242) -> (appended path=w245:path)
        n113 = Build Path(base path=w245, name or relative path=w244) -> (appended path=w234:path)
        n114 = invoke class="App" method="Library.Create"(error in=w232) -> (error out=w237:errorcluster, "Create Library"=w236:refnum<vi>)  [unwired: 3 in, 2 out]
        n115 = invoke class="Library" method="Save"(reference=w236, error in=w237, "Path"=w234) -> (reference out=w235:refnum<vi>, error out=w233:errorcluster)  [unwired: 1 in, 2 out]
        n116 = Bundle By Name(cluster=w238, "System Explorer Library"=w235) -> (w239:T1)
      }
      frame "PC-System Explorer - Add folders and VIs to library" {
        # "On the diagram of Main VI, replace the stub subVI for Load Help File.vi with the actual new VI."
        # "Add virtual folders and all VIs to <CD> System Explorer.lvlib"
        n117 = property class="Consolidated_CD"(reference=w250) -> ("Project Root"=w249:path, "Accessors:CD Template"=w248:refnum<class "NIVS_CD Template.lvclass">)  [unwired: 1 in, 2 out]
        n118 = property class="CD Template"(reference=w248) -> ("Accessors:Extra Page Names"=w247:string[])  [unwired: 1 in, 2 out]
        n119 = call "System Explorer - Add content to System Explorer library.vi"("error in (no error)"=w267, "Extra Page Names"=w247, "Project Root"=w249, "CD Wizard - Internal Data"=w265) -> ("error out"=w266:errorcluster, "System Explorer Main VI"=w256:path, "Load Help File VI"=w255:path)  [unwired: 5 in]
        n120 = Open VI Reference(vi path=w256, error in (no error)=w266) -> (vi reference=w262:refnum<vi>, error out=w264:errorcluster)  [unwired: 4 in]
        n121 = call <vilib>:"TRef Find Object By Label.vi"("Label"="Load Help File_stub.vi", "Traverse Target"=TRef_TravTarget."BD", "error in (no error)"=w264, "Class Name"="SubVI", "VI Ref"=w262) -> ("error out"=w263:errorcluster, "Found Obj Ref"=w257:refnum<vi>, "dup VI Ref"=w253:refnum<vi>)  [unwired: 3 in, 1 out]
        n122 = invoke class="GObj" method="Replace"(reference=w257, error in=w263, "Path"=w255) -> (error out=w258:errorcluster)  [unwired: 3 in, 5 out]
        n123 = invoke class="VI" method="Save.Instrument"(reference=w253, error in=w258) -> (reference out=w251:refnum<vi>, error out=w254:errorcluster)  [unwired: 4 in, 4 out]
        n124 = Close Reference(reference=w251, error in (no error)=w254) -> (error out=w252:errorcluster)
      }
      frame "PC-Engine - Create folder and copy the RT Template" {
        # "Create a new Engine folder on the file system and copy the RT Driver VI for the chosen custom device."
        n125 = property class="Consolidated_CD"(reference=w272) -> ("Accessors:CD Template"=w269:refnum<class "NIVS_CD Template.lvclass">, "Project Name"=w271:string, "Project Root"=w270:path)  [unwired: 1 in, 2 out]
        n126 = call-dynamic "Create Engine Folder and Copy RT Template.vi"("error in (no error)"=w275, "Project Root"=w270, "Project Name"=w271, "CD Template"=w269) -> ("error out"=w274:errorcluster)  [unwired: 7 in]
      }
      frame "PC-Engine - Create library" {
        # "Create the library for the Engine components."
        n127 = property class="Consolidated_CD"(reference=w279) -> ("Project Name"=w278:string, "Project Root"=w277:path)  [unwired: 1 in, 2 out]
        n128 = call-poly "Constants Main.vi"("Action"=CD_Engine_lvlib."LibraryFolderName") -> ("Output"=w290:string)  [unwired: 10 in]
        n129 = call-poly "Constants Main.vi"("Action"=CD_Engine_lvlib."LibraryFileName") -> ("Output"=w291:string)  [unwired: 10 in]
        n130 = Format Into String(format string=w291, w278) -> (resulting string=w292:string)  [unwired: 2 in, 1 out]
        n131 = Build Path(base path=w277, name or relative path=w290) -> (appended path=w293:path)
        n132 = Build Path(base path=w293, name or relative path=w292) -> (appended path=w281:path)
        n133 = invoke class="App" method="Library.Create"(error in=w280) -> (error out=w285:errorcluster, "Create Library"=w284:refnum<vi>)  [unwired: 3 in, 2 out]
        n134 = invoke class="Library" method="Save"(reference=w284, error in=w285, "Path"=w281) -> (reference out=w282:refnum<vi>, error out=w283:errorcluster)  [unwired: 1 in, 2 out]
        n135 = Bundle By Name(cluster=w287, "Engine Library"=w282) -> (w286:T1)
      }
      frame "PC-Engine - Add virtual folders and VIs to library" {
        # "Add all virtual folders and template VIs to the Engine library"
        n136 = property class="Consolidated_CD"(reference=w299) -> ("Accessors:CD Template"=w297:refnum<class "NIVS_CD Template.lvclass">, "Project Root"=w296:path, "Project Name"=w295:string)  [unwired: 1 in, 2 out]
        n137 = call-dynamic "Add content to Engine library.vi"("Project Name"=w295, "error in (no error)"=w301, "Project Root"=w296, "CD Wizard - Internal Data"=w298, "CD Template"=w297) -> ("error out"=w300:errorcluster)  [unwired: 6 in]
      }
      frame "PC-XML - Create and change file" {
        # "Create the XML file and add it to the project tree"
        n138 = call "XML - Create XML file.vi"("error in (no error)"=w306, "Consolidated_CD"=w303, "CD Wizard - Internal Data"=w304) -> ("error out"=w305:errorcluster)  [unwired: 7 in, 1 out]
      }
      frame "PC-Help - Copy HTML Files" {
        w322 = "Main"
        w337 = "OPTIONS" ("section")
        # "Note: We only copy the files here, the get added to the project in the \"Write New Project File\" case since the project doesn't exist (to add the folder to) until that case."
        # "Copy all of the HTML template files to the new help directory, and configure Build CHM file."
        n139 = property class="Consolidated_CD"(reference=w312) -> ("Project Name"=w311:string, "Project Root"=w310:path, "Accessors:CD Template"=w309:refnum<class "NIVS_CD Template.lvclass">)  [unwired: 1 in, 2 out]
        n140 = property class="CD Template"(reference=w309) -> ("Accessors:Extra Page Names"=w308:string[])  [unwired: 1 in, 2 out]
        n141 = Build Path(base path=w310, name or relative path=path "Help") -> (appended path=w321:path)
        n142 = call <vilib>:"Check if File or Folder Exists.vi"("error in (no error)"=w324, "path"=w321) -> ("error out"=w330:errorcluster, "file or folder exists?"=w344:bool, "dup path"=w345:path)  [unwired: 7 in]
        n143 = case shown="False" w344 {
          tunnel: w345 -> [w348 w352]
          tunnel: [w348 w351] -> w316
          tunnel: [w347 w350] -> w331
          tunnel: w330 -> [w347 w349]
          frame False {
          }
          frame True {
            n144 = Delete(path (use dialog)=w352, entire hierarchy (F)=TRUE, error in=w349) -> (deleted path=w351:path, error out=w350:errorcluster)  [unwired: 2 in, 1 out]
          }
        }
        n145 = Build Array (concatenate)(w322, w308) -> (w315:string[])
        n146 = Concatenate Strings("HTML Help Source\\" ("string"), w322, ".htm" ("string")) -> (w326:string)
        n147 = Create Folder(path (use dialog)=w316, error in=w331) -> (created path=w318:path, error out=w317:errorcluster)  [unwired: 1 in, 1 out]
        n148 = call "Call HTML Help Generation Functions Async.vi"("error in (no error)"=w317, "Extra Page Names"=w315, "Destination Base Path"=w318) -> ("error out"=w314:errorcluster, "Destination Base Path Out (dup)"=w313:path)  [unwired: 7 in]
        n149 = Build Path(base path=w318, name or relative path="Build CHM.cfg") -> (appended path=w328:path)
        n150 = call <vilib>:"Open Config Data.vi"("error in (no error)"=w314, "configuration file path"=w328) -> ("error out"=w343:errorcluster, "refnum"=w342:T13)  [unwired: 7 in, 1 out]
        n151 = call-poly <vilib>:"Write Key.vi"("section"=w337, "error in (no error)"=w343, "value"=w311, "key"="Title", "refnum"=w342) -> ("error out"=w340:errorcluster, "refnum out"=w339:T13)  [unwired: 4 in, 1 out]
        n152 = call-poly <vilib>:"Write Key.vi"("section"=w337, "error in (no error)"=w340, "value"=w326, "key"="Default Topic", "refnum"=w339) -> ("error out"=w336:errorcluster, "refnum out"=w334:T13)  [unwired: 4 in, 1 out]
        n153 = call-poly <vilib>:"Write Key.vi"("section"=w337, "error in (no error)"=w336, "value"=w313, "key"="Base Path", "refnum"=w334) -> ("error out"=w335:errorcluster, "refnum out"=w333:T13)  [unwired: 4 in, 1 out]
        n154 = call <vilib>:"Close Config Data.vi"("error in (no error)"=w335, "refnum"=w333) -> ("error out"=w323:errorcluster)  [unwired: 8 in, 1 out]
      }
      frame "Project - Read project file content" {
        w365 = -1  # Read all lines
        w364 = T12."open"  # operation
        w363 = enum16{"read/write", "read-only", "write-only"}."read-only"  # access
        # "Open the project file and read the complete content."
        n155 = call-poly "Constants Main.vi"("Action"=Common."ProjectTemplatePathAndName") -> ("Output"=w356:string)  [unwired: 10 in]
        n156 = String To Path(string=w356) -> (path=w357:path)
        n157 = Open/Create/Replace File(file path (use dialog)=w357, error in=w354, operation (0:open)=w364, access (0:read/write)=w363) -> (refnum out=w361:refnum<file>, error out=w362:errorcluster)  [unwired: 3 out]
        n158 = Read from Text File(file (use dialog)=w361, count=w365, error in=w362) -> (refnum out=w355:refnum<file>, text=w359:string[], error out=w360:errorcluster)  [unwired: 2 out]
        n159 = Close File(refnum=w355) -> ()  [unwired: 1 in, 2 out]
      }
      frame "Project - Edit Utility section" {
        # "Edit the entries for the utility folder. Also added CHM pre build action entries"
        n160 = call-poly "Constants Main.vi"("Action"=Utility_folder."Utility.FolderName") -> ("Output"=w372:string)  [unwired: 10 in]
        n161 = call-poly "Constants Main.vi"("Action"=Utility_folder."Utility.Copy .llb to NI VeriStand dir.FileName") -> ("Output"=w373:string)  [unwired: 10 in]
        n162 = call-poly "Constants Main.vi"("Action"=Utility_folder."Utility.LLB Pre Build.FilePathAndName") -> ("Output"=w370:string)  [unwired: 10 in]
        n163 = String To Path(string=w370) -> (path=w369:path)
        n164 = Strip Path(path=w369) -> (name=w368:string)  [unwired: 1 out]
        n165 = for "For Iterate over each line and change the placeholders for the Utility entries." {
          tunnel: w378 -> [w390] mode=indexing
          shift-right: [w386] -> w376
          shift-left: w367 -> [w388]
          tunnel: [w384] -> w377 mode=indexing
          tunnel: w373 -> [w389]
          tunnel: w372 -> [w387]
          tunnel: w368 -> [w380]
          w382 = TRUE  # ignore case?
          w383 = TRUE  # replace all?
          w393 = "%CopyLLBtoNIVSFileName%"  # search
          w395 = "%UtilityFolderName%"  # search
          # "CHM Build VI as pre-build action"
          # "Copy .LLB to NI VeriStand dir.vi"
          # "Utility"
          n166 = Search and Replace String(replace all?=w383, case sensitive?=w382, input string=w390, search string=w395, replace string=w387, error in=w388) -> (result string=w394:string, error out=w392:errorcluster)  [unwired: 2 in, 2 out]
          n167 = Search and Replace String(replace all?=w383, case sensitive?=w382, input string=w394, search string=w393, replace string=w389, error in=w392) -> (result string=w385:string, error out=w391:errorcluster)  [unwired: 2 in, 2 out]
          n168 = Search and Replace String(replace all?=w383, case sensitive?=w382, input string=w385, search string="%CHMPreBuild%" ("result string"), replace string=w380, error in=w391) -> (result string=w384:string, error out=w386:errorcluster)  [unwired: 2 in, 2 out]
        }
      }
      frame "Project - Edit XML section" {
        # "Edit the Name and Path for the XML file."
        n169 = property class="Consolidated_CD"(reference=w398) -> ("Project Name"=w397:string, "Accessors:CD Template"=w396:refnum<class "NIVS_CD Template.lvclass">)  [unwired: 1 in, 2 out]
        n170 = call "XML - Get XML file name.vi"("CD Template"=w396, "CD Name"=w397) -> ("XML file name"=w400:string)  [unwired: 9 in]
        n171 = for "Iterate over each line and change the placeholder for the XML file name." {
          tunnel: w403 -> [w411] mode=indexing
          shift-right: [w410] -> w404
          shift-left: w399 -> [w406]
          tunnel: [w409] -> w402 mode=indexing
          tunnel: w400 -> [w405]
          w407 = TRUE  # ignore case?
          w408 = TRUE  # replace all?
          w412 = "%XMLCustomDeviceFileName%"  # search
          n172 = Search and Replace String(replace all?=w408, case sensitive?=w407, input string=w411, search string=w412, replace string=w405, error in=w406) -> (result string=w409:string, error out=w410:errorcluster)  [unwired: 2 in, 2 out]
        }
      }
      frame "Project - Edit Engine Library section" {
        # "Edit the entries for the Engine Library (Library name and folder name)"
        n173 = property class="Consolidated_CD"(reference=w414) -> ("Project Name"=w413:string)  [unwired: 1 in, 2 out]
        n174 = call "Change Engine Library Placeholders in project.vi"("error in (no error)"=w418, "Project Name"=w413, "Project file content in"=w415) -> ("error out"=w417:errorcluster, "Project file content out"=w419:string[])  [unwired: 7 in]
      }
      frame "Project - Edit Shared Library section" {
        # "Edit the entries for the Shared Library (Library name and folder name)"
        n175 = property class="Consolidated_CD"(reference=w421) -> ("Project Name"=w420:string)  [unwired: 1 in, 2 out]
        n176 = call-poly "Constants Main.vi"("Action"=CD_Shared_lvlib."LibraryFileName") -> ("Output"=w429:string)  [unwired: 10 in]
        n177 = call-poly "Constants Main.vi"("Action"=CD_Shared_lvlib."LibraryFolderName") -> ("Output"=w425:string)  [unwired: 10 in]
        n178 = call-poly "Constants Main.vi"("Action"=CD_Shared_lvlib."Shared.FolderName") -> ("Output"=w424:string)  [unwired: 10 in]
        n179 = Format Into String(format string=w429, w420) -> (resulting string=w426:string)  [unwired: 2 in, 1 out]
        n180 = for "Iterate over each line and change the placeholder for the Shared Library file and folder name." {
          tunnel: w427 -> [w448] mode=indexing
          shift-right: [w441] -> w432
          shift-left: w422 -> [w447]
          tunnel: [w442] -> w433 mode=indexing
          tunnel: w426 -> [w436]
          tunnel: w425 -> [w435]
          tunnel: w424 -> [w434]
          w439 = "%SharedLibrarySubfolderName%"  # search
          w445 = "%SharedLibraryFolderName%"  # search
          w437 = TRUE  # ignore case?
          w438 = TRUE  # replace all?
          w449 = "%SharedLibraryFileName%"  # search
          # "Shared"
          # "Shared"
          # "<CD> Shared.lvlib"
          n181 = Search and Replace String(replace all?=w438, case sensitive?=w437, input string=w448, search string=w449, replace string=w436, error in=w447) -> (result string=w446:string, error out=w444:errorcluster)  [unwired: 2 in, 2 out]
          n182 = Search and Replace String(replace all?=w438, case sensitive?=w437, input string=w446, search string=w445, replace string=w435, error in=w444) -> (result string=w443:string, error out=w440:errorcluster)  [unwired: 2 in, 2 out]
          n183 = Search and Replace String(replace all?=w438, case sensitive?=w437, input string=w443, search string=w439, replace string=w434, error in=w440) -> (result string=w442:string, error out=w441:errorcluster)  [unwired: 2 in, 2 out]
        }
      }
      frame "Project - Edit System Explorer Library section" {
        # "Edit the entries for the System Explorer Library (Library name and folder name)"
        n184 = property class="Consolidated_CD"(reference=w451) -> ("Project Name"=w450:string)  [unwired: 1 in, 2 out]
        n185 = call-poly "Constants Main.vi"("Action"=CD_System_Explorer_lvlib."LibraryFileName") -> ("Output"=w458:string)  [unwired: 10 in]
        n186 = Format Into String(format string=w458, w450) -> (resulting string=w461:string)  [unwired: 2 in, 1 out]
        n187 = call-poly "Constants Main.vi"("Action"=CD_System_Explorer_lvlib."System Explorer.FolderName") -> ("Output"=w463:string)  [unwired: 10 in]
        n188 = call-poly "Constants Main.vi"("Action"=CD_System_Explorer_lvlib."LibraryFolderName") -> ("Output"=w462:string)  [unwired: 10 in]
        n189 = for "Iterate over each line and change the placeholder for the System Explorer Library file and folder name." {
          tunnel: w454 -> [w478] mode=indexing
          shift-right: [w470] -> w456
          shift-left: w452 -> [w477]
          tunnel: [w471] -> w455 mode=indexing
          tunnel: w461 -> [w466]
          tunnel: w462 -> [w465]
          tunnel: w463 -> [w464]
          w467 = "%SystemExplorerSubfolderName%"  # search
          w475 = "%SystemExplorerLibraryFolderName%"  # search
          w469 = TRUE  # ignore case?
          w468 = TRUE  # replace all?
          w479 = "%SystemExplorerLibraryFileName%"  # search
          n190 = Search and Replace String(replace all?=w468, case sensitive?=w469, input string=w478, search string=w479, replace string=w466, error in=w477) -> (result string=w476:string, error out=w474:errorcluster)  [unwired: 2 in, 2 out]
          n191 = Search and Replace String(replace all?=w468, case sensitive?=w469, input string=w476, search string=w475, replace string=w465, error in=w474) -> (result string=w472:string, error out=w473:errorcluster)  [unwired: 2 in, 2 out]
          n192 = Search and Replace String(replace all?=w468, case sensitive?=w469, input string=w472, search string=w467, replace string=w464, error in=w473) -> (result string=w471:string, error out=w470:errorcluster)  [unwired: 2 in, 2 out]
        }
      }
      frame "Project - Edit Custom Device Name" {
        # "Edit the Custom Device name"
        n193 = property class="Consolidated_CD"(reference=w481) -> ("Project Name"=w480:string)  [unwired: 1 in, 2 out]
        n194 = for "Iterate over each line and change the placeholder for the Custom Device name." {
          tunnel: w483 -> [w493] mode=indexing
          shift-right: [w488] -> w485
          shift-left: w486 -> [w489]
          tunnel: [w492] -> w484 mode=indexing
          tunnel: w480 -> [w487]
          w490 = TRUE  # ignore case?
          w491 = TRUE  # replace all?
          w494 = "%CustomDeviceName%"  # search
          # "<CD>"
          n195 = Search and Replace String(replace all?=w491, case sensitive?=w490, input string=w493, search string=w494, replace string=w487, error in=w489) -> (result string=w492:string, error out=w488:errorcluster)  [unwired: 2 in, 2 out]
        }
      }
      frame "Project - Edit System Explorer LLB Name" {
        # "Edit the name for the System Explorer LLB."
        n196 = property class="Consolidated_CD"(reference=w496) -> ("Project Name"=w495:string)  [unwired: 1 in, 2 out]
        n197 = call-poly "Constants Main.vi"("Action"=Build_Spec_System_Explorer."Destinations.LLBFileName") -> ("Output"=w503:string)  [unwired: 10 in]
        n198 = Format Into String(format string=w503, w495) -> (resulting string=w500:string)  [unwired: 2 in, 1 out]
        n199 = for "Iterate over each line and change the placeholder for the System Explorer LLB." {
          tunnel: w500 -> [w510]
          tunnel: w499 -> [w508] mode=indexing
          tunnel: [w507] -> w498 mode=indexing
          shift-right: [w506] -> w504
          shift-left: w497 -> [w509]
          w505 = "%SystemExplorerLLBFileName%"  # search
          w511 = TRUE  # ignore case?
          w512 = TRUE  # replace all?
          # "<CD> Configuration.llb"
          n200 = Search and Replace String(replace all?=w512, case sensitive?=w511, input string=w508, search string=w505, replace string=w510, error in=w509) -> (result string=w507:string, error out=w506:errorcluster)  [unwired: 1 in, 3 out]
        }
      }
      frame "Project - Edit Engine LLB OS dependent file name" {
        n201 = property class="Consolidated_CD"(reference=w514) -> ("Project Name"=w513:string)  [unwired: 1 in, 2 out]
        n202 = call-poly "Constants Main.vi"("Action"=Build_Spec_Engine."Destinations.LLBLinux64FileName") -> ("Output"=w524:string)  [unwired: 10 in]
        n203 = call-poly "Constants Main.vi"("Action"=Build_Spec_Engine."Destinations.LLBLinuxARMFileName") -> ("Output"=w525:string)  [unwired: 10 in]
        n204 = call-poly "Constants Main.vi"("Action"=Build_Spec_Engine."Destinations.LLBPharlapFileName") -> ("Output"=w530:string)  [unwired: 10 in]
        n205 = call-poly "Constants Main.vi"("Action"=Build_Spec_Engine."Destinations.LLBWindowsFileName") -> ("Output"=w535:string)  [unwired: 10 in]
        n206 = call-poly "Constants Main.vi"("Action"=Build_Spec_Engine."Destinations.LLBVxWorksFileName") -> ("Output"=w531:string)  [unwired: 10 in]
        n207 = Format Into String(format string=w524, w513) -> (resulting string=w518:string)  [unwired: 2 in, 1 out]
        n208 = Format Into String(format string=w525, w513) -> (resulting string=w519:string)  [unwired: 2 in, 1 out]
        n209 = Format Into String(format string=w535, w513) -> (resulting string=w522:string)  [unwired: 2 in, 1 out]
        n210 = Format Into String(format string=w531, w513) -> (resulting string=w521:string)  [unwired: 2 in, 1 out]
        n211 = Format Into String(format string=w530, w513) -> (resulting string=w520:string)  [unwired: 2 in, 1 out]
        n212 = Build Array(w522, w521, w520, w519, w518) -> (w517:string[])
        n213 = for {
          shift-right: [w540] -> w527
          shift-left: w515 -> [w541]
          tunnel: w528 -> [w537] mode=indexing
          tunnel: w517 -> [w538]
          tunnel: [w536] -> w516 mode=indexing
          n214 = for {
            shift-right: [w549] -> w540
            shift-left: w541 -> [w548]
            shift-right: [w545] -> w536
            shift-left: w537 -> [w544]
            tunnel: string[] ["%EngineLLBWindowsFileName%", "%EngineLLBVxWorksFileName%", "%EngineLLBPharlapFileName%", "%EngineLLBLinuxARMFileName%", "%EngineLLBLinux64FileName%"] -> [w543] mode=indexing
            tunnel: w538 -> [w542] mode=indexing
            w546 = TRUE  # ignore case?
            w547 = TRUE  # replace all?
            n215 = Search and Replace String(replace all?=w547, case sensitive?=w546, input string=w544, search string=w543, replace string=w542, error in=w548) -> (result string=w545:string, error out=w549:errorcluster)  [unwired: 1 in, 3 out]
          }
        }
      }
      frame "Project - Write new project file" {
        # "Create new file and write the project file content into it."
        n216 = property class="Consolidated_CD"(reference=w552) -> ("Project Name"=w551:string, "Project Root"=w550:path)  [unwired: 1 in, 2 out]
        n217 = call-poly "Constants Main.vi"("Action"=Common."ProjectName") -> ("Output"=w576:string)  [unwired: 10 in]
        n218 = Format Into String(format string=w576, w551) -> (resulting string=w587:string)  [unwired: 2 in, 1 out]
        n219 = Build Path(base path=w550, name or relative path=w587) -> (appended path=w582:path)
        n220 = Open/Create/Replace File(file path (use dialog)=w582, error in=w553, operation (0:open)=T12."replace or create") -> (refnum out=w584:refnum<file>, error out=w583:errorcluster)  [unwired: 3 in, 1 out]
        n221 = Write to Text File(file (use dialog)=w584, text=w579, error in=w583) -> (refnum out=w581:refnum<file>, error out=w580:errorcluster)  [unwired: 2 out]
        n222 = Close File(refnum=w581, error in=w580) -> (path=w577:path, error out=w575:errorcluster)
        n223 = invoke class="App" method="Project.Open"(error in=w575, "Path"=w577) -> (error out=w570:errorcluster, "Project:Open"=w569:refnum<vi>)  [unwired: 2 in, 2 out]
        n224 = Build Path(base path=w550, name or relative path=path "Help") -> (appended path=w563:path)
        n225 = property class="Project"(reference=w569, error in=w570) -> (reference out=w568:refnum<vi>, error out=w566:errorcluster, "My Computer"=w567:refnum<vi>)
        n226 = invoke class="TargetItem" method="AddItem"(reference=w567, error in=w566, "Name"="Placeholder", "Path"=path "", "Type"="Folder") -> (reference out=w556:refnum<vi>, error out=w573:errorcluster, "AddItem"=w572:refnum<vi>)  [unwired: 1 in, 3 out]
        n227 = invoke class="ProjectItem" method="Convert to Auto-populating Folder"(reference=w572, error in=w573, "Path"=w563) -> (reference out=w558:refnum<vi>, error out=w554:errorcluster)  [unwired: 1 in, 2 out]
        n228 = Close Reference(reference=w558) -> (error out=w557:errorcluster)  [unwired: 1 in]
        n229 = invoke class="Project" method="Open Window"(reference=w568, error in=w554) -> (reference out=w555:refnum<vi>, error out=w559:errorcluster)  [unwired: 1 in, 1 out]
        n230 = Close Reference(reference=w556, error in (no error)=w557) -> ()  [unwired: 1 out]
        n231 = invoke class="Project" method="Save"(reference=w555, error in=w559) -> (reference out=w561:refnum<vi>, error out=w562:errorcluster)  [unwired: 2 in, 2 out]
        n232 = Close Reference(reference=w561, error in (no error)=w562) -> (error out=w560:errorcluster)
      }
    }
  }
  "error out" <- w6
